vi "Open.vi"(0 "resources":T18[](array[typedef]), 1 "hardware configuration":T4, 2 "option string":string="sample_rate=3.072G", 5 "7902 bitfile download":bool=TRUE, 7 "3620 bitfile download":bool, 9 "run cal & sync":bool=TRUE, 11 "error in":errorcluster, 14 "legacy init":bool) -> (4 "session out":T6[](array[typedef]) {"rx baseband session"."3630 session"."Address Space" items=["VXI/VME A16"=1, "VXI/VME A24"=2, "VXI/VME A32"=3, "VXI/VME A64"=4, "PXI Memory Allocations"=9, "PXI Configuration"=10, "PXI BAR0"=11, "PXI BAR1"=12, "PXI BAR2"=13, "PXI BAR3"=14, "PXI BAR4"=15, "PXI BAR5"=16]; "tx baseband session"."3610 session"."Address Space" items=["VXI/VME A16"=1, "VXI/VME A24"=2, "VXI/VME A32"=3, "VXI/VME A64"=4, "PXI Memory Allocations"=9, "PXI Configuration"=10, "PXI BAR0"=11, "PXI BAR1"=12, "PXI BAR2"=13, "PXI BAR3"=14, "PXI BAR4"=15, "PXI BAR5"=16]}, 6 "detected mmWave adapters":T1[](array[typedef]) {"detected mmWave adapters"."serial number" format="%.0x"}, 15 "error out":errorcluster)   [LabVIEW 2019, in "mmWave HW Control.lvlib"]
uses:
  mmWave HW Control.lvlib
  Low-level/TypeDefs/Resources.ctl
  <vilib>/userdefined/High Color/nirio_resource_hc.ctl
  Low-level/TypeDefs/Session.ctl
  <instrlib>/niMmWave/ni3620/Config/v1/Host/Public/High-Level/niMmWave Session.ctl
  <instrlib>/_niInstr/Register Bus/v0/Host/Public/Register Bus Session.ctl
  <instrlib>/_niInstr/Register Bus/v0/Host/Private/Session Data.ctl
  <instrlib>/niMmWave/ni3620/Config/v1/Host/Public/Typedefs/Board Information.ctl
  <instrlib>/niMmWave/ni3620/Config/v1/Host/Public/Typedefs/Hardware Revision.ctl
  <instrlib>/niMmWave/ni3620/Config/v1/Host/Public/Typedefs/Gain Mapping.ctl
  <instrlib>/niMmWave/ni3620/Config/v1/Host/Public/Typedefs/Correction Data.ctl
  <instrlib>/niMmWave/ni3620/Config/v1/Host/Public/Typedefs/Opera Characterization.ctl
  <instrlib>/niMmWave/ni3620/Config/v1/Host/Public/Corrections/Typedefs/Opera Characterization Main Header.ctl
  <instrlib>/niMmWave/ni3620/Config/v1/Host/Public/Corrections/Typedefs/Opera IF Board Information.ctl
  <instrlib>/niMmWave/ni3620/Config/v1/Host/Public/Corrections/Typedefs/Opera Characterization Instance Header.ctl
  <instrlib>/niMmWave/ni3620/Config/v1/Host/Public/Corrections/Typedefs/Opera Characterization Device Data Header.ctl
  <instrlib>/niMmWave/ni3620/Config/v1/Host/Public/Corrections/Typedefs/Opera LO Characterization Data Header.ctl
  <instrlib>/niMmWave/ni3620/Config/v1/Host/Public/Corrections/Typedefs/Opera IF Board Characterization Data Header.ctl
  <instrlib>/niMmWave/ni3620/Config/v1/Host/Public/Corrections/Typedefs/Opera Characterization Device Data.ctl
  <instrlib>/niMmWave/ni3620/Config/v1/Host/Public/Corrections/Typedefs/Opera LO2 Board Characterization Data.ctl
  <instrlib>/niMmWave/ni3620/Config/v1/Host/Public/Corrections/Typedefs/Opera LO Characterization Data.ctl
  <instrlib>/niMmWave/ni3620/Config/v1/Host/Public/Corrections/Typedefs/Opera IF Board Characterization Data.ctl
  <instrlib>/niMmWave/ni3620/Config/v1/Host/Public/Corrections/Typedefs/Opera IQ Impairment Data.ctl
  <instrlib>/niMmWave/ni3620/Config/v1/Host/Public/Typedefs/mmWave Adapter Session Data.ctl
  <instrlib>/niMmWave/ni3620/Config/v1/Host/Public/Typedefs/mmWave Adapter Data.ctl
  <instrlib>/niMmWave/ni3620/Config/v1/Host/Public/Typedefs/mmWave Adapter 2.ctl
  <instrlib>/niMmWave/ni3620/Config/v1/Shared/Typedefs/Subsystem ID.ctl
  <instrlib>/niMmWave/ni3620/Config/v1/Host/Public/Typedefs/mmWave Adapter Channel Information.ctl
  <instrlib>/niMmWave/ni3620/Config/v1/Host/Public/Typedefs/Temperature Coefficients.ctl
  <instrlib>/niMmWave/ni3620/Config/v1/Host/Public/Typedefs/mmWave Characterization.ctl
  <instrlib>/niMmWave/ni3620/Config/v1/Host/Public/Corrections/Typedefs/mmWave Characterization Main Header.ctl
  <instrlib>/niMmWave/ni3620/Config/v1/Host/Public/Corrections/Typedefs/mmWave Characterization Instance Header.ctl
  <instrlib>/niMmWave/ni3620/Config/v1/Host/Public/Typedefs/Session Cache.ctl
  <instrlib>/niMmWave/ni3620/Config/v1/Host/Public/Typedefs/LO2 settings cache.ctl
  <instrlib>/niMmWave/ni3620/Config/v1/Host/Public/Typedefs/LO2 source.ctl
  <instrlib>/niMmWave/ni3620/Config/v1/Host/Public/Typedefs/Desired and Coerced.ctl
  <instrlib>/niMmWave/ni3620/Config/v1/Host/Public/Typedefs/Export cache.ctl
  <instrlib>/niMmWave/ni3620/Config/v1/Host/Public/Typedefs/Path cache.ctl
  <instrlib>/niMmWave/ni3620/Config/v1/Host/Public/Typedefs/Daughterboard Type.ctl
  <instrlib>/niMmWave/ni3620/Config/v1/Host/Public/Typedefs/LO1 settings cache.ctl
  <instrlib>/niMmWave/ni3620/Config/v1/Host/Public/Typedefs/LO1 Source.ctl
  <instrlib>/niMmWave/ni3620/Config/v1/Host/Public/Typedefs/mmWave export cache.ctl
  <instrlib>/niMmWave/ni3620/Config/v1/Host/Private/Board/LO2/LO2 Board Configuration Cache.ctl
  <instrlib>/niMmWave/ni3620/Config/v1/Host/Public/Typedefs/reference clock routing settings.ctl
  <instrlib>/niMmWave/ni3620/Config/v1/Host/Public/Typedefs/LO2 routing settings.ctl
  <instrlib>/niMmWave/ni3620/Config/v1/Host/Private/Board/LO1/LO1 Board Configuration Cache.ctl
  <instrlib>/niMmWave/ni3620/Config/v1/Host/Public/Typedefs/LO1 source settings.ctl
  <instrlib>/niMmWave/ni3620/Config/v1/Host/Public/Typedefs/LO1 export settings.ctl
  <instrlib>/niMmWave/ni3620/Config/v1/Host/Public/Typedefs/LO1 mmWave settings.ctl
  Low-level/TypeDefs/Tx Baseband Session.ctl
  <instrlib>/niMmWave/ni3610 and ni3630/controls/public/Main Settings.ctl
  <vilib>/Instr/_visa.llb/VISA Register Access Address Space.ctl
  <instrlib>/niMmWave/ni3610 and ni3630/controls/public/Register Adresses.ctl
  <instrlib>/niMmWave/ni3610 and ni3630/controls/public/Base Card Type.ctl
  <instrlib>/niMmWave/ni3610 and ni3630/controls/private/IQ Card Revision.ctl
  <instrlib>/niMmWave/ni3610 and ni3630/controls/public/Board Capability.ctl
  Low-level/TypeDefs/Blank FPGA Reference.ctl
  Low-level/TypeDefs/Rx Baseband Session.ctl
  Low-level/TypeDefs/Hardware Configuration.ctl
  Low-level/TypeDefs/Direction.ctl
  Low-level/TypeDefs/Gain Ranging.ctl
  Low-level/TypeDefs/PXI Trigger Bus Info.ctl
  Low-level/TypeDefs/Detected mmWave Adapters.ctl
  Low-level/TypeDefs/mmWave Adapter Information.ctl
  <instrlib>/niMmWave/ni3620/Config/v1/Host/Public/Typedefs/Rx IF signal source.ctl
  <instrlib>/niMmWave/ni3620/Config/v1/Host/Public/Typedefs/Tx IF signal destination.ctl
  Low-level/TypeDefs/RX FPGA Reference.ctl
  Low-level/TypeDefs/TX FPGA Reference.ctl
  Low-level/Calibration/Hardware Settings.ctl
  <vilib>/Utility/error.llb/Error Cluster From Error Code.vi
  <vilib>/rvi/errors/niLvFpgaAdjustHostInterfaceError.vi
  <vilib>/rvi/interface/nirviReadWriteControl/nirviReadWriteControl.xnode
  <instrlib>/niMmWave/ni3620/Config/v1/Host/niMmWave Config v1 Host.lvlib
  <instrlib>/_niInstr/Register Bus/v0/Host/niInstr Register Bus v0 Host.lvlib
  <instrlib>/niMmWave/ni3610 and ni3630/ni3610_and_ni3630_Driver_Lib.lvlib
  <instrlib>/niMmWave/ni3620/Config/v1/Shared/niMmWave Config v1 Shared.lvlib
  NiFpgaLv.dll
  <vilib>/rvi/interface/Simulation/niFpgaSimulationCallBeginRW.vi
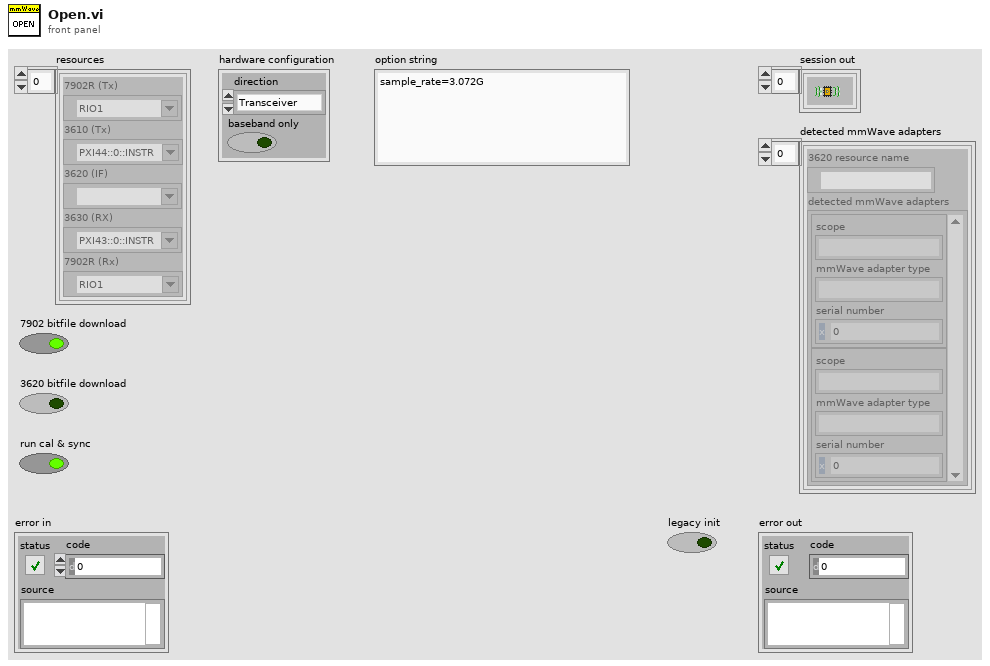
[diagram p1: front panel]
types:
  T1 = typedef "Detected mmWave Adapters.ctl" = cluster{"3620 resource name":T2, "detected mmWave adapters":T3[]}
  T2 = typedef "nirio_resource_hc.ctl" = tag
  T3 = typedef "mmWave Adapter Information.ctl" = cluster{"scope":string, "mmWave adapter type":string, "serial number":u64}
  T4 = typedef "Hardware Configuration.ctl" = cluster{"direction":T5, "baseband only":bool}
  T5 = typedef "Direction.ctl" = enum16{"Transceiver", "Receiver", "Transmitter"}
  T6 = typedef "Session.ctl" = cluster{"3620 session":refnum<queue>, "tx baseband session":T7, "rx baseband session":T15, "tx gain (dB)":dbl, "rx gain (dB)":dbl, "hardware configuration":T4, "gain ranging":T16[], "pxi trigger bus information":T17}
  T7 = typedef "Tx Baseband Session.ctl" = cluster{"3610 session":T8, "7902 reference":T14}
  T8 = typedef "ni3610_and_ni3630_Driver_Lib.lvlib/Main Settings.ctl" = cluster{"VISA resource name":refnum<visa-resource-name>, "Address Space":T9, "window_offset":u32, "register_addresses":T10, "required_MM_fpga_version":cluster{"signature":u32, "hardware":u32, "current revision":u32, "oldest revision":u32}, "CPLD Oldest Compat Version ":cluster{"hardware":u32, "CPLD firmware":u32}, "MM_FPGA_image_location":string, "is_init":bool, "card_type":T11, "DacLmkConfigFileName":string, "AdcLmkConfigFileName":string, "AdcConfigFileName":string, "DacConfigFileName_RevA":string, "DacConfigFileName_RevB":string, "Mulde hardware revision":u8, "bypass DAC PLL\n":bool, "IQ Card Revision":T12, "board capability":T13}
  T9 = typedef "VISA Register Access Address Space.ctl" = u16
  T10 = typedef "ni3610_and_ni3630_Driver_Lib.lvlib/Register Adresses.ctl" = cluster{"MM based Registers":cluster{"Revision":u32, "OldestCompatRev":u32, "signature":u32, "scratch":u32, "LedControl":u32, "BoardHwRev":u32, "BoardControl":u32, "ThermalStatus":u32, "BasebandStatus":u32, "BasebandControl":u32, "BasebandAuxSetup":u32, "BasebandAuxStatus":u32, "LmkSyncOutSetup":u32, " AdcSyncOutSetup":u32, " InjSyncOutSetup":u32, " PxiTrig0OutSetup":u32, " PxiTrig1OutSetup":u32, " PxiTrig2OutSetup":u32, " PxiTrig3OutSetup":u32, " PxiTrig4OutSetup":u32, " PxiTrig5OutSetup":u32, " PxiTrig6OutSetup":u32, " PxiTrig7OutSetup":u32}, "CPLD based Registers":cluster{"SlaveSignature":u32, "SlaveRevision":u32, "SlaveOldestCompatRev":u32, "SlaveScratch":u32, "SlaveSetup":u32, "SlaveStatus":u32, "IDacReg_offset":u32, "LMKRegGrp0_offset":u32, "QDacReg_offset":u32, "BrdTempSensorVal":u32, "TempSensorPowerDown":u32, "GPIOReg_offset":u32, "IAdcReg_offset":u32, "QAdcReg_offset":u32, "LMKRegGrp1_offset":u32, "QadcTempSensorVal":u32, "IadcTempSensorVal":u32, "RevisionReg":u32, "VcxoReg":u32, "CpldStatusReg":u32, "PowerReg":u32, "VBiasEnReg":u32, "ExtRefOeReg":u32, "QdacCtrlReg":u32, "QdacStatusReg":u32, "IdacCtrlReg":u32, "IdacStatusReg":u32, "QdacJtagIn":u32, "QdacJtagOut":u32, "IdacJtagIn":u32, "IdacJtagOut":u32, "IqDcSetupReg":u32, "QadcStatusReg":u32, "IadcStatusReg":u32, "BrdSetupReg":u32, "IqDcRevisionReg":u32, "PllStatusReg":u32, "EndpointScratchReg":u32, "AdcSyncCfgReg":u32, "IqCardOpampReg":u32}, "CPLD Register Offset":u32, "MM  Register Offset":u32, " PxiTrig0OutSetup":u32}
  T11 = typedef "ni3610_and_ni3630_Driver_Lib.lvlib/Base Card Type.ctl" = enum16{"unspecified", "ADC", "DAC"}
  T12 = typedef "ni3610_and_ni3630_Driver_Lib.lvlib/IQ Card Revision.ctl" = enum16{"RevA", "RevB", "RevC", "RevD"}
  T13 = typedef "ni3610_and_ni3630_Driver_Lib.lvlib/Board Capability.ctl" = cluster{"baseband sync":enum16{"no baseband sync", "baseband sync"}}
  T14 = typedef "Blank FPGA Reference.ctl" = refnum<k20>
  T15 = typedef "Rx Baseband Session.ctl" = cluster{"3630 session":T8, "7902 reference":T14}
  T16 = typedef "Gain Ranging.ctl" = cluster{"gain ranging active scope":string, "gain ranging stream session":refnum<k20>}
  T17 = typedef "PXI Trigger Bus Info.ctl" = cluster{"chassis resource name":refnum<visa-resource-name>, "7902R (TX)":i16, "3610 (TX)":i16, "3620 (IF)":i16, "3630 (RX)":i16, "7902R (RX)":i16}
  T18 = typedef "Resources.ctl" = cluster{"7902R (Tx)":T2, "3610 (Tx)":refnum<visa-resource-name>, "3620 (IF)":T2, "3630 (RX)":refnum<visa-resource-name>, "7902R (Rx)":T2}
  T19 = cluster{"scope":string, "mmWave Adapter type":string, "Serial Number":u64}
  T20 = typedef "niMmWave Config v1 Host.lvlib/Tx IF signal destination.ctl" = enum16{"IF Output", "IF Loopback", "Cal Output", "Disabled"}
  T21 = typedef "niMmWave Config v1 Host.lvlib/Rx IF signal source.ctl" = enum16{"IF Input", "IF Loopback", "External Cal Input", "Internal Cal Input"}
  T22 = typedef "TX FPGA Reference.ctl" = refnum<k20>
  T23 = typedef "RX FPGA Reference.ctl" = refnum<k20>
  T24 = typedef "Hardware Settings.ctl" = cluster{"RX IF Gain":dbl, "TX IF Gain":dbl}
  T25 = enum16{"TClk Trigger", "TClk Measure", "ADC Sync Injection", "Tx JESD Sync", "Rx JESD Sync", "Tx ADC Sync Injection", "Tx Master10k_Reset"}[]
  T26 = typedef "niMmWave Config v1 Host.lvlib/mmWave Adapter Information.ctl" = cluster{"scope":string, "mmWave adapter type":string, "board information":T27}
  T27 = typedef "niMmWave Config v1 Host.lvlib/Board Information.ctl" = cluster{"product code":u16, "hardware revision":T28, "serial number":u64}
  T28 = typedef "niMmWave Config v1 Host.lvlib/Hardware Revision.ctl" = enum16{"Unknown", "A", "B", "C", "D", "E", "F", "G", "H", "I", "J"}
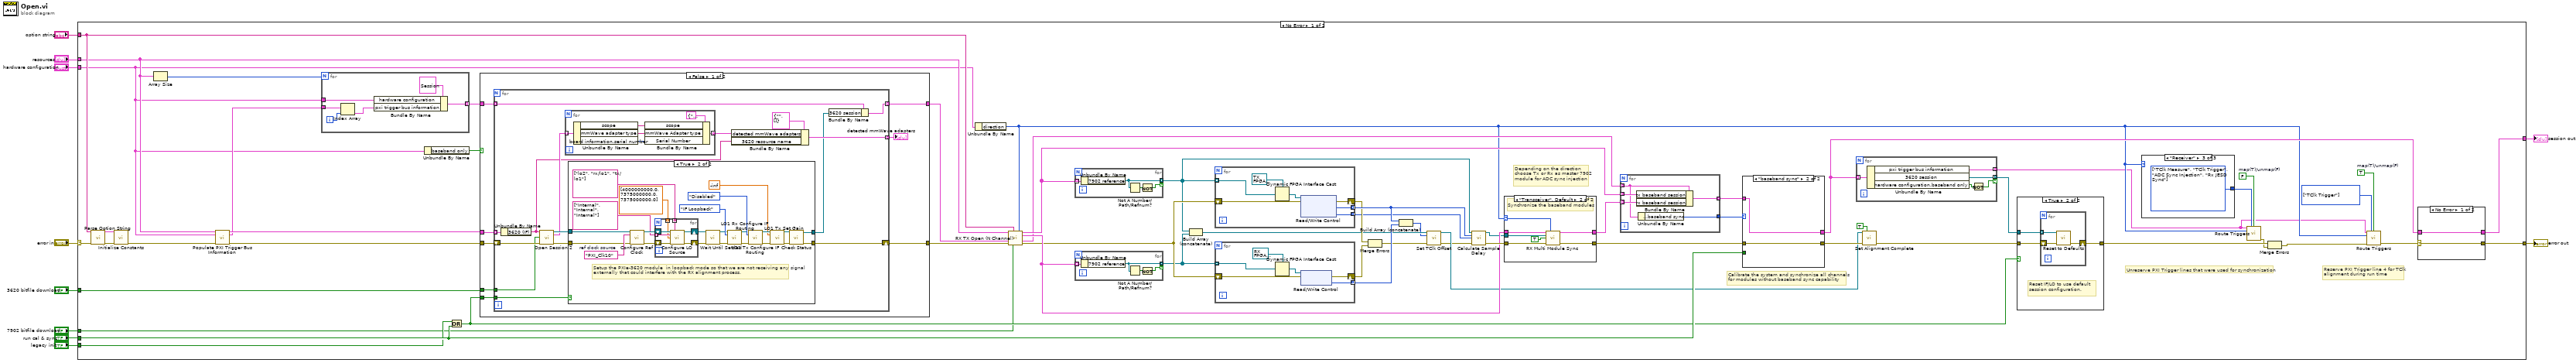
[diagram p0: block diagram]
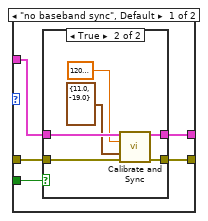
[diagram p4: hidden frame]
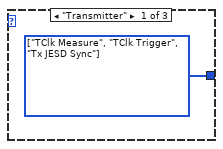
[diagram p6: hidden frame]
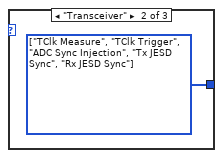
[diagram p7: hidden frame]
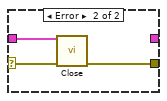
[diagram p9: hidden frame]
diagram:
  n1 = case shown="No Error" "error in" {
    selector: "error in" -> [w46 w209]
    tunnel: "resources" -> [w40 _]
    tunnel: [w51 _] -> w9
    tunnel: [w55 w209] -> w8
    tunnel: "7902 bitfile download" -> [w39 _]
    tunnel: "hardware configuration" -> [w32 _]
    tunnel: "run cal & sync" -> [w62 _]
    tunnel: "3620 bitfile download" -> [w65 _]
    tunnel: "legacy init" -> [w61 _]
    tunnel: "option string" -> [w41 _]
    frame No Error {
      w25 = TRUE  # map(T)/unmap(F)
      w26 = T25 [enum."TClk Trigger"] items=["TClk Trigger", "TClk Measure", "ADC Sync Injection", "Tx JESD Sync", "Rx JESD Sync", "Tx ADC Sync Injection", "Tx Master10k_Reset"] ("route for")
      w63 = FALSE  # map(T)/unmap(F)
      # "Reserve PXI Trigger line 4 for TClk\nalignment during run time"
      # "Depending on the direction\nchoose Tx or Rx as master 7902\nmodule for ADC sync injection"
      # "Unreserve PXI Trigger lines that were used for synchronization"
      # "Calibrate the system and synchronize all channels\nfor modules without baseband sync capability"
      n2 = call "Parse Option String.vi"("option string"=w41, "error in"=w46) -> ("option name/value pairs"=w45:cluster{"option":string, "value":string}[], "error out"=w44:errorcluster)  [unwired: 12 in]
      n3 = call "Initialize Constants.vi"("option name/value pairs"=w45, "error in"=w44) -> ("error out"=w43:errorcluster)  [unwired: 13 in]
      n4 = Array Size(array=w40) -> (size(s)=w60:i32)
      n5 = call "Populate PXI Trigger Bus Information.vi"("hardware resources [channel]"=w40, "hardware setup"=w32, "error in (no error)"=w43) -> ("hardware resources out"=w58:T18[], "pxi trigger bus segment information [channel]"=w52:T17[], "error out"=w31:errorcluster)  [unwired: 10 in]
      n6 = for {
        N: w60 -> [_]
        tunnel: w52 -> [w135]
        tunnel: w32 -> [w137]
        tunnel: [w136] -> w59 mode=indexing
        i -> [w134]
        n7 = Index Array(array=w135, index=w134) -> (element=w133:T17)
        n8 = Bundle By Name(cluster=T6 {"3620 session"=refnum, "tx baseband session"={"3610 session"={"VISA resource name"="", "Address Space"=1, "window_offset"=0, "register_addresses"={"MM based Registers"={"Revision"=0, "OldestCompatRev"=0, "signature"=0, "scratch"=0, "LedControl"=0, "BoardHwRev"=0, "BoardControl"=0, "ThermalStatus"=0, "BasebandStatus"=0, "BasebandControl"=0, "BasebandAuxSetup"=0, "BasebandAuxStatus"=0, "LmkSyncOutSetup"=0, " AdcSyncOutSetup"=0, " InjSyncOutSetup"=0, " PxiTrig0OutSetup"=0, " PxiTrig1OutSetup"=0, " PxiTrig2OutSetup"=0, " PxiTrig3OutSetup"=0, " PxiTrig4OutSetup"=0, " PxiTrig5OutSetup"=0, " PxiTrig6OutSetup"=0, " PxiTrig7OutSetup"=0}, "CPLD based Registers"={"SlaveSignature"=0, "SlaveRevision"=0, "SlaveOldestCompatRev"=0, "SlaveScratch"=0, "SlaveSetup"=0, "SlaveStatus"=0, "IDacReg_offset"=0, "LMKRegGrp0_offset"=0, "QDacReg_offset"=0, "BrdTempSensorVal"=0, "TempSensorPowerDown"=0, "GPIOReg_offset"=0, "IAdcReg_offset"=0, "QAdcReg_offset"=0, "LMKRegGrp1_offset"=0, "QadcTempSensorVal"=0, "IadcTempSensorVal"=0, "RevisionReg"=0, "VcxoReg"=0, "CpldStatusReg"=0, "PowerReg"=0, "VBiasEnReg"=0, "ExtRefOeReg"=0, "QdacCtrlReg"=0, "QdacStatusReg"=0, "IdacCtrlReg"=0, "IdacStatusReg"=0, "QdacJtagIn"=0, "QdacJtagOut"=0, "IdacJtagIn"=0, "IdacJtagOut"=0, "IqDcSetupReg"=0, "QadcStatusReg"=0, "IadcStatusReg"=0, "BrdSetupReg"=0, "IqDcRevisionReg"=0, "PllStatusReg"=0, "EndpointScratchReg"=0, "AdcSyncCfgReg"=0, "IqCardOpampReg"=0}, "CPLD Register Offset"=0, "MM  Register Offset"=0, " PxiTrig0OutSetup"=0}, "required_MM_fpga_version"={"signature"=0, "hardware"=0, "current revision"=0, "oldest revision"=0}, "CPLD Oldest Compat Version "={"hardware"=0, "CPLD firmware"=0}, "MM_FPGA_image_location"="", "is_init"=FALSE, "card_type"=enum."ADC", "DacLmkConfigFileName"="", "AdcLmkConfigFileName"="", "AdcConfigFileName"="", "DacConfigFileName_RevA"="", "DacConfigFileName_RevB"="", "Mulde hardware revision"=0, "bypass DAC PLL\n"=FALSE, "IQ Card Revision"=enum."RevA", "board capability"={"baseband sync"=enum."no baseband sync"}}, "7902 reference"=refnum}, "rx baseband session"={"3630 session"={"VISA resource name"="", "Address Space"=1, "window_offset"=0, "register_addresses"={"MM based Registers"={"Revision"=0, "OldestCompatRev"=0, "signature"=0, "scratch"=0, "LedControl"=0, "BoardHwRev"=0, "BoardControl"=0, "ThermalStatus"=0, "BasebandStatus"=0, "BasebandControl"=0, "BasebandAuxSetup"=0, "BasebandAuxStatus"=0, "LmkSyncOutSetup"=0, " AdcSyncOutSetup"=0, " InjSyncOutSetup"=0, " PxiTrig0OutSetup"=0, " PxiTrig1OutSetup"=0, " PxiTrig2OutSetup"=0, " PxiTrig3OutSetup"=0, " PxiTrig4OutSetup"=0, " PxiTrig5OutSetup"=0, " PxiTrig6OutSetup"=0, " PxiTrig7OutSetup"=0}, "CPLD based Registers"={"SlaveSignature"=0, "SlaveRevision"=0, "SlaveOldestCompatRev"=0, "SlaveScratch"=0, "SlaveSetup"=0, "SlaveStatus"=0, "IDacReg_offset"=0, "LMKRegGrp0_offset"=0, "QDacReg_offset"=0, "BrdTempSensorVal"=0, "TempSensorPowerDown"=0, "GPIOReg_offset"=0, "IAdcReg_offset"=0, "QAdcReg_offset"=0, "LMKRegGrp1_offset"=0, "QadcTempSensorVal"=0, "IadcTempSensorVal"=0, "RevisionReg"=0, "VcxoReg"=0, "CpldStatusReg"=0, "PowerReg"=0, "VBiasEnReg"=0, "ExtRefOeReg"=0, "QdacCtrlReg"=0, "QdacStatusReg"=0, "IdacCtrlReg"=0, "IdacStatusReg"=0, "QdacJtagIn"=0, "QdacJtagOut"=0, "IdacJtagIn"=0, "IdacJtagOut"=0, "IqDcSetupReg"=0, "QadcStatusReg"=0, "IadcStatusReg"=0, "BrdSetupReg"=0, "IqDcRevisionReg"=0, "PllStatusReg"=0, "EndpointScratchReg"=0, "AdcSyncCfgReg"=0, "IqCardOpampReg"=0}, "CPLD Register Offset"=0, "MM  Register Offset"=0, " PxiTrig0OutSetup"=0}, "required_MM_fpga_version"={"signature"=0, "hardware"=0, "current revision"=0, "oldest revision"=0}, "CPLD Oldest Compat Version "={"hardware"=0, "CPLD firmware"=0}, "MM_FPGA_image_location"="", "is_init"=FALSE, "card_type"=enum."ADC", "DacLmkConfigFileName"="", "AdcLmkConfigFileName"="", "AdcConfigFileName"="", "DacConfigFileName_RevA"="", "DacConfigFileName_RevB"="", "Mulde hardware revision"=0, "bypass DAC PLL\n"=FALSE, "IQ Card Revision"=enum."RevA", "board capability"={"baseband sync"=enum."no baseband sync"}}, "7902 reference"=refnum}, "tx gain (dB)"=0.0, "rx gain (dB)"=0.0, "hardware configuration"={"direction"=enum."Transceiver", "baseband only"=FALSE}, "gain ranging"=[], "pxi trigger bus information"={"chassis resource name"="", "7902R (TX)"=0, "3610 (TX)"=0, "3620 (IF)"=0, "3630 (RX)"=0, "7902R (RX)"=0}} ("session"), "hardware configuration"=w137, "pxi trigger bus information"=w133) -> (w136:T6)
      }
      n9 = Unbundle By Name(w32) -> ("baseband only"=w64:bool)
      n10 = Or(x=w61, y=w62) -> (x .or. y?=w57:bool)
      n11 = case shown="False" w64 {
        tunnel: w31 -> [w77 w132]
        tunnel: [w76 w132] -> w42
        tunnel: w65 -> [w75 _]
        tunnel: w57 -> [w73 _]
        tunnel: w59 -> [w72 w131]
        tunnel: [w71 w131] -> w34
        tunnel: w58 -> [w70 _]
        frame False {
          n12 = for {
            tunnel: w70 -> [w92] mode=indexing
            shift-right: [w90] -> w76
            shift-left: w77 -> [w91]
            tunnel: w75 -> [w89]
            tunnel: [w85] -> w74 mode=indexing
            tunnel: w73 -> [w81]
            tunnel: w72 -> [w80] mode=indexing
            tunnel: [w78] -> w71 mode=indexing
            n13 = Unbundle By Name(w92) -> ("3620 (IF)"=w82:T2)
            n14 = call <instrlib>:"Open Session 2.vi"("resource name"=w82, "force bitfile download"=w89, "error in"=w91) -> ("session out"=w88:refnum<queue>, "mmWave adapters information"=w83:T26[], "error out"=w87:errorcluster)  [unwired: 10 in]
            n15 = for {
              tunnel: w83 -> [w98] mode=indexing
              tunnel: [w93] -> w86 mode=indexing
              n16 = Unbundle By Name(w98) -> ("scope"=w96:string, "mmWave adapter type"=w95:string, "board information.serial number"=w94:u64)
              n17 = Bundle By Name(cluster=T19 {"scope"="", "mmWave Adapter type"="", "Serial Number"=0} ("HeadInfo"), "scope"=w96, "mmWave Adapter type"=w95, "Serial Number"=w94) -> (w93:T19)
            }
            n18 = case shown="True" w81 {
              tunnel: w88 -> [w100 w112]
              tunnel: w87 -> [w99 w111]
              tunnel: [w100 w103] -> w79
              tunnel: [w99 w101] -> w90
              frame False {
              }
              frame True {
                w119 = "PXI_Clk10"  # ref clock source
                # "Setup the PXIe-3620 module  in loopback mode so that we are not receiving any signal externally that could interfere with the RX alignment process."
                n19 = call <instrlib>:"Configure Ref Clock.vi"("session in"=w112, "ref clock source"=w119, "error in"=w111) -> ("session out"=w121:refnum<queue>, "error out"=w120:errorcluster)  [unwired: 11 in]
                n20 = for {
                  shift-right: [w128] -> w109
                  shift-left: w121 -> [w130]
                  shift-right: [w127] -> w110
                  shift-left: w120 -> [w129]
                  tunnel: string[] ["Internal", "Internal", "Internal"] -> [w126] mode=indexing
                  tunnel: string[] ["lo2", "rx/lo1", "tx/lo1"] -> [w124] mode=indexing
                  tunnel: dbl[] [4000000000.0, 7375000000.0, 7375000000.0] -> [w125] mode=indexing
                  n21 = call <instrlib>:"Configure LO Source.vi"("session in"=w130, "scope"=w124, "LO source"=w126, "frequency (Hz)"=w125, "error in"=w129) -> ("session out"=w128:refnum<queue>, "error out"=w127:errorcluster)  [unwired: 9 in]
                }
                n22 = call <instrlib>:"Wait Until Settled.vi"("session in"=w109, "error in"=w110) -> ("session out"=w107:refnum<queue>, "error out"=w108:errorcluster)  [unwired: 12 in]
                n23 = call <instrlib>:"LO1 Rx Configure IF Routing.vi"("session in"=w107, "IF signal source"=Rx_IF_signal_source."IF Loopback", "error in"=w108) -> ("session out"=w106:refnum<queue>, "error out"=w105:errorcluster)  [unwired: 11 in]
                n24 = call <instrlib>:"LO1 Tx Configure IF Routing.vi"("session in"=w106, "IF signal destination"=Tx_IF_signal_destination."Disabled", "error in"=w105) -> ("session out"=w114:refnum<queue>, "error out"=w115:errorcluster)  [unwired: 11 in]
                n25 = call <instrlib>:"LO1 Tx Set Gain.vi"("session in"=w114, "gain (dB)"=-inf, "error in"=w115) -> ("session out"=w104:refnum<queue>, "error out"=w102:errorcluster)  [unwired: 10 in, 1 out]
                n26 = call <instrlib>:"Check Status.vi"("session in"=w104, "error in"=w102) -> ("session out"=w103:refnum<queue>, "error out"=w101:errorcluster)  [unwired: 12 in]
              }
            }
            n27 = Bundle By Name(cluster=T1 {"3620 resource name"="", "detected mmWave adapters"=[]} ("Cluster"), "detected mmWave adapters"=w86, "3620 resource name"=w82) -> (w85:T1)
            n28 = Bundle By Name(cluster=w80, "3620 session"=w79) -> (w78:T6)
          }
          "detected mmWave adapters" <- w74
        }
        frame True {
        }
      }
      n29 = Unbundle By Name(w32) -> ("direction"=w24:T5)
      n30 = call "RX TX Open (N Channel).vi"("resources"=w40, "option string"=w41, "direction"=w24, "session in"=w34, "error in"=w42, "force download"=w39) -> ("tx baseband session out"=w36:T7[], "rx baseband session out"=w38:T15[], "session out"=w33:T6[], "error out"=w37:errorcluster)  [unwired: 6 in]
      n31 = for {
        tunnel: w36 -> [w155] mode=indexing
        tunnel: [w154] -> w13 mode=indexing if=w152
        n32 = Unbundle By Name(w155) -> ("7902 reference"=w154:T14)
        n33 = Not A Number/Path/Refnum?(number/path/refnum=w154) -> (NaN/Path/Refnum?=w153:bool)
        n34 = Not(x=w153) -> (.not. x?=w152:bool)
      }
      n35 = for {
        tunnel: w38 -> [w159] mode=indexing
        tunnel: [w158] -> w12 mode=indexing if=w156
        n36 = Unbundle By Name(w159) -> ("7902 reference"=w158:T14)
        n37 = Not A Number/Path/Refnum?(number/path/refnum=w158) -> (NaN/Path/Refnum?=w157:bool)
        n38 = Not(x=w157) -> (.not. x?=w156:bool)
      }
      n39 = Build Array (concatenate)(w13, w12) -> (w18:T14[])
      n40 = for {
        tunnel: w13 -> [w145] mode=indexing
        shift-right: [w141] -> w19
        shift-left: w37 -> [w142]
        tunnel: [w140] -> w22 mode=indexing
        tunnel: [w139] -> w14 mode=indexing
        n41 = Dynamic FPGA Interface Cast(Session In=T22 refnum ("Refnum in"), Type=w145) -> (Session Out=w143:T22)
        n42 = xnode "Read/Write Control"("FPGA VI Reference In"=w143, "error in"=w142) -> ("error out"=w141:errorcluster, "tclk value"=w140:u16, "sysref value"=w139:u8)  [unwired: 1 out]
      }
      n43 = for {
        tunnel: w12 -> [w147] mode=indexing
        shift-right: [w149] -> w20
        shift-left: w37 -> [w150]
        tunnel: [w146] -> w21 mode=indexing
        n44 = Dynamic FPGA Interface Cast(Session In=T23 refnum ("fpga reference"), Type=w147) -> (Session Out=w151:T23)
        n45 = xnode "Read/Write Control"("FPGA VI Reference In"=w151, "error in"=w150) -> ("error out"=w149:errorcluster, "tclk value"=w146:u16)  [unwired: 1 out]
      }
      n46 = Merge Errors(w19, w20) -> (w17:errorcluster)
      n47 = Build Array (concatenate)(w22, w21) -> (w15:u16[])
      n48 = call "Set TClk Offset.vi"("fpga reference in"=w18, "tclk trigger value"=w15, "error in"=w17) -> ("fpga reference out"=w30:T14[], "error out"=w16:errorcluster)  [unwired: 11 in]
      n49 = call "Calculate Sample Delay.vi"("fpga reference in"=w13, "tclk values"=w22, "sysref values"=w14, "error in"=w16) -> ("fpga reference out"=w29:T14[], "error out"=w69:errorcluster)  [unwired: 10 in]
      n50 = case shown="\"Transceiver\", Default" w24 {
        selector: w24 -> [_ w198]
        tunnel: w69 -> [w196 w203]
        tunnel: [w196 w202] -> w67
        tunnel: [w195 w201] -> w66
        tunnel: w38 -> [w195 w200]
        tunnel: w29 -> [_ w199]
        frame "Transmitter" {
        }
        frame "Transceiver", Default {
          # "Synchronize the baseband modules"
          n51 = call "RX Multi Module Sync.vi"("rx baseband session in"=w200, "direction"=w198, "fpga reference in"=w199, "absolute delay"=TRUE, "error in"=w203) -> ("rx baseband session out"=w201:T15[], "error out"=w202:errorcluster)  [unwired: 8 in, 1 out]
        }
      }
      n52 = for {
        tunnel: w36 -> [w206] mode=indexing
        tunnel: [w208] -> w68 mode=indexing
        tunnel: w66 -> [w207] mode=indexing
        tunnel: w33 -> [w205] mode=indexing
        tunnel: [w204] -> w11
        n53 = Bundle By Name(cluster=w205, "tx baseband session"=w206, "rx baseband session"=w207) -> (w208:T6)
        n54 = Unbundle By Name(w205) -> ("tx baseband session.3610 session.board capability.baseband sync"=w204:enum16{"no baseband sync", "baseband sync"})
      }
      n55 = case shown="\"baseband sync\"" w11 {
        tunnel: w68 -> [w164 w173]
        tunnel: w67 -> [w163 w174]
        tunnel: w62 -> [w162 _]
        tunnel: [w161 w173] -> w50
        tunnel: [w160 w174] -> w48
        frame "no baseband sync", Default {
          n56 = case shown="True" w162 {
            tunnel: [w166 w172] -> w161
            tunnel: [w165 w171] -> w160
            tunnel: w164 -> [w166 w170]
            tunnel: w163 -> [w165 w169]
            frame False {
            }
            frame True {
              n57 = call "Calibrate and Sync.vi"("session in"=w170, "IF frequency (Hz)"=12000000000.0 ("x"), "hardware settings"=T24 {"RX IF Gain"=11.0, "TX IF Gain"=-19.0}, "error in"=w169) -> ("session out"=w172:T6[], "error out"=w171:errorcluster)  [unwired: 10 in]
            }
          }
        }
        frame "baseband sync" {
        }
      }
      n58 = for {
        tunnel: w50 -> [w182] mode=indexing
        tunnel: [w181] -> w23 mode=indexing
        tunnel: [w180] -> w56 mode=indexing if=w179
        n59 = Unbundle By Name(w182) -> ("pxi trigger bus information"=w181:T17, "3620 session"=w180:refnum<queue>, "hardware configuration.baseband only"=w178:bool)
        n60 = Not(x=w178) -> (.not. x?=w179:bool)
      }
      n61 = call "Set Alignment Complete.vi"("fpga ref in"=w30, "alignment complete"=TRUE, "error in"=w48) -> ("error out"=w47:errorcluster)  [unwired: 11 in, 1 out]
      n62 = case shown="True" w57 {
        tunnel: w56 -> [_ w186]
        tunnel: w47 -> [w183 w185]
        tunnel: [w183 w184] -> w54
        frame False {
        }
        frame True {
          # "Reset IF/LO to use default session configuration."
          n63 = for {
            tunnel: w186 -> [w189] mode=indexing
            shift-right: [w187] -> w184
            shift-left: w185 -> [w188]
            n64 = call <instrlib>:"Reset to Defaults.vi"("session in"=w189, "error in"=w188) -> ("error out"=w187:errorcluster)  [unwired: 12 in, 1 out]
          }
        }
      }
      n65 = case shown="\"Receiver\"" w24 {
        tunnel: [w175 w176 w177] -> w35
        frame "Transmitter" {
          w175 = T25 [enum."TClk Measure", enum."TClk Trigger", enum."Tx JESD Sync"] items=["TClk Trigger", "TClk Measure", "ADC Sync Injection", "Tx JESD Sync", "Rx JESD Sync", "Tx ADC Sync Injection", "Tx Master10k_Reset"] ("route for")
        }
        frame "Transceiver" {
          w176 = T25 [enum."TClk Measure", enum."TClk Trigger", enum."ADC Sync Injection", enum."Tx JESD Sync", enum."Rx JESD Sync"] items=["TClk Trigger", "TClk Measure", "ADC Sync Injection", "Tx JESD Sync", "Rx JESD Sync", "Tx ADC Sync Injection", "Tx Master10k_Reset"] ("route for")
        }
        frame "Receiver" {
          w177 = T25 [enum."TClk Measure", enum."TClk Trigger", enum."ADC Sync Injection", enum."Rx JESD Sync"] items=["TClk Trigger", "TClk Measure", "ADC Sync Injection", "Tx JESD Sync", "Rx JESD Sync", "Tx ADC Sync Injection", "Tx Master10k_Reset"] ("route for")
        }
      }
      n66 = call "Route Triggers.vi"("pxi trigger bus configuration [channel]"=w23, "route for"=w35, "map(T)/unmap(F)"=w63, "Direction"=w24) -> ("error out"=w53:errorcluster)  [unwired: 11 in]
      n67 = Merge Errors(w54, w53) -> (w28:errorcluster)
      n68 = call "Route Triggers.vi"("pxi trigger bus configuration [channel]"=w23, "route for"=w26, "map(T)/unmap(F)"=w25, "Direction"=w24, "error in"=w28) -> ("error out"=w27:errorcluster)  [unwired: 10 in]
      n69 = case shown="No Error" w27 {
        selector: w27 -> [w191 w193]
        tunnel: w50 -> [w190 w194]
        tunnel: [w191 w192] -> w55
        tunnel: [w190 _] -> w51
        frame No Error {
        }
        frame Error {
          n70 = call "Close.vi"("session"=w194, "error in"=w193) -> ("error out"=w192:errorcluster)  [unwired: 13 in]
        }
      }
    }
    frame Error {
    }
  }
  "error out" <- w8
  "session out" <- w9
